vi "String Time to Time Stamp.vi"(8 "error in (no error)":errorcluster, 11 "input TimeStamp string":string(combo)) -> (0 "error out":errorcluster, 3 "Time Stamp":timestamp)   [LabVIEW 2021]
doc: "2021-01-01 00:00:01.000 \nstring format to Time Stamp format"
panel:
  # "13:55:33.345 09/27/2021"
  # "2021-09-27 16:55:33.345"
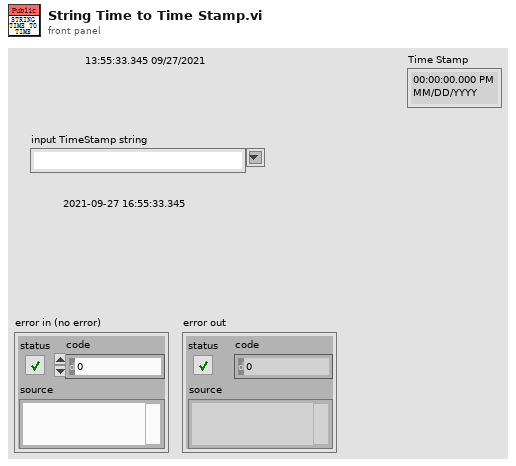
[diagram p1: front panel]
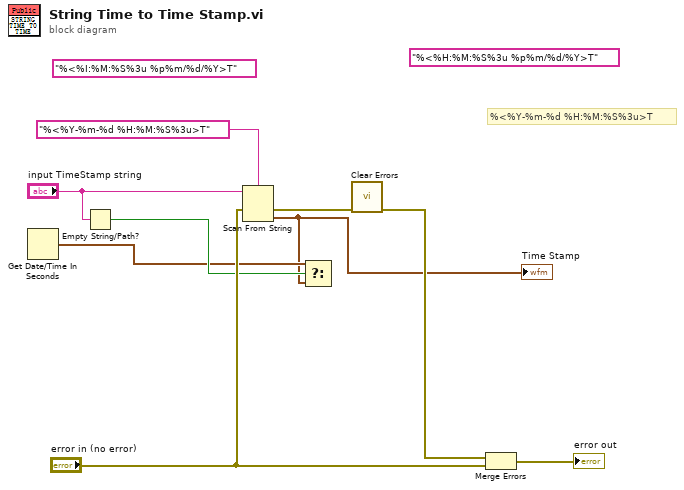
[diagram p0: block diagram]
diagram:
  (unwired) "%<%H:%M:%S%3u %p%m/%d/%Y>T" ("format string")
  (unwired) "%<%I:%M:%S%3u %p%m/%d/%Y>T" ("format string")
  # "%<%Y-%m-%d %H:%M:%S%3u>T"
  n1 = Get Date/Time In Seconds() -> (seconds since 1Jan1904=w3:timestamp)
  n2 = Empty String/Path?(string/path="input TimeStamp string") -> (empty?=w4:bool)
  n3 = Scan From String(format string="%<%Y-%m-%d %H:%M:%S%3u>T", input string="input TimeStamp string", error in="error in (no error)") -> (error out=w8:errorcluster, output 1=w1:timestamp)  [unwired: 2 in, 2 out]
  "Time Stamp" <- w1
  n4 = Select(t=w3, s=w4, f=w1) -> ()  [unwired: 1 out]
  n5 = call <vilib>:"Clear Errors.vi"("error in (no error)"=w8) -> ("error out"=w2:errorcluster)  [unwired: 5 in, 1 out]
  n6 = Merge Errors(w2, "error in (no error)") -> (→"error out":errorcluster)
